vi "Main.vi"() -> ()   [LabVIEW 2023]
panel:
  in  "Marker_Size":string
  out "Color Box 5":u32(colorbox)
  out "Color Box 4":u32(colorbox)
  out "Color Box 3":u32(colorbox)
  out "Color Box 2":u32(colorbox)
  out "Color Box":u32(colorbox)
  out "error out":errorcluster
  out "Corner color":u32(colorbox)
  out "Colors traces":string
  out "standard output":string
  out "CLUT":u32[](array[numeric])
  in  "Path":path
  in  "style of points":string
  out "PnG picture":picture
  out "Pixmap vraie couleurs":u32[](array[numeric])
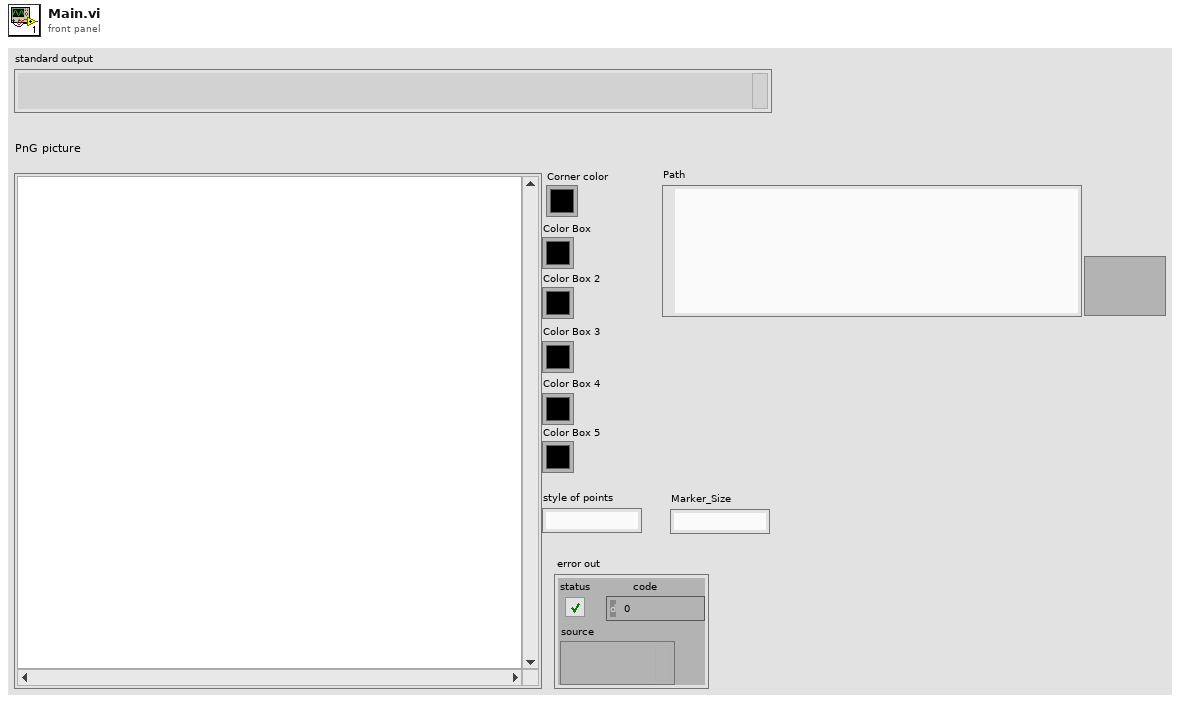
[diagram p1: front panel]
types:
  T1 = cluster{"[0]":u32, "[1]":u32, "[2]":u32, "[3]":u32, "[4]":u32, "[5]":u32, "[6]":u32, "[7]":u32, "[8]":u32}
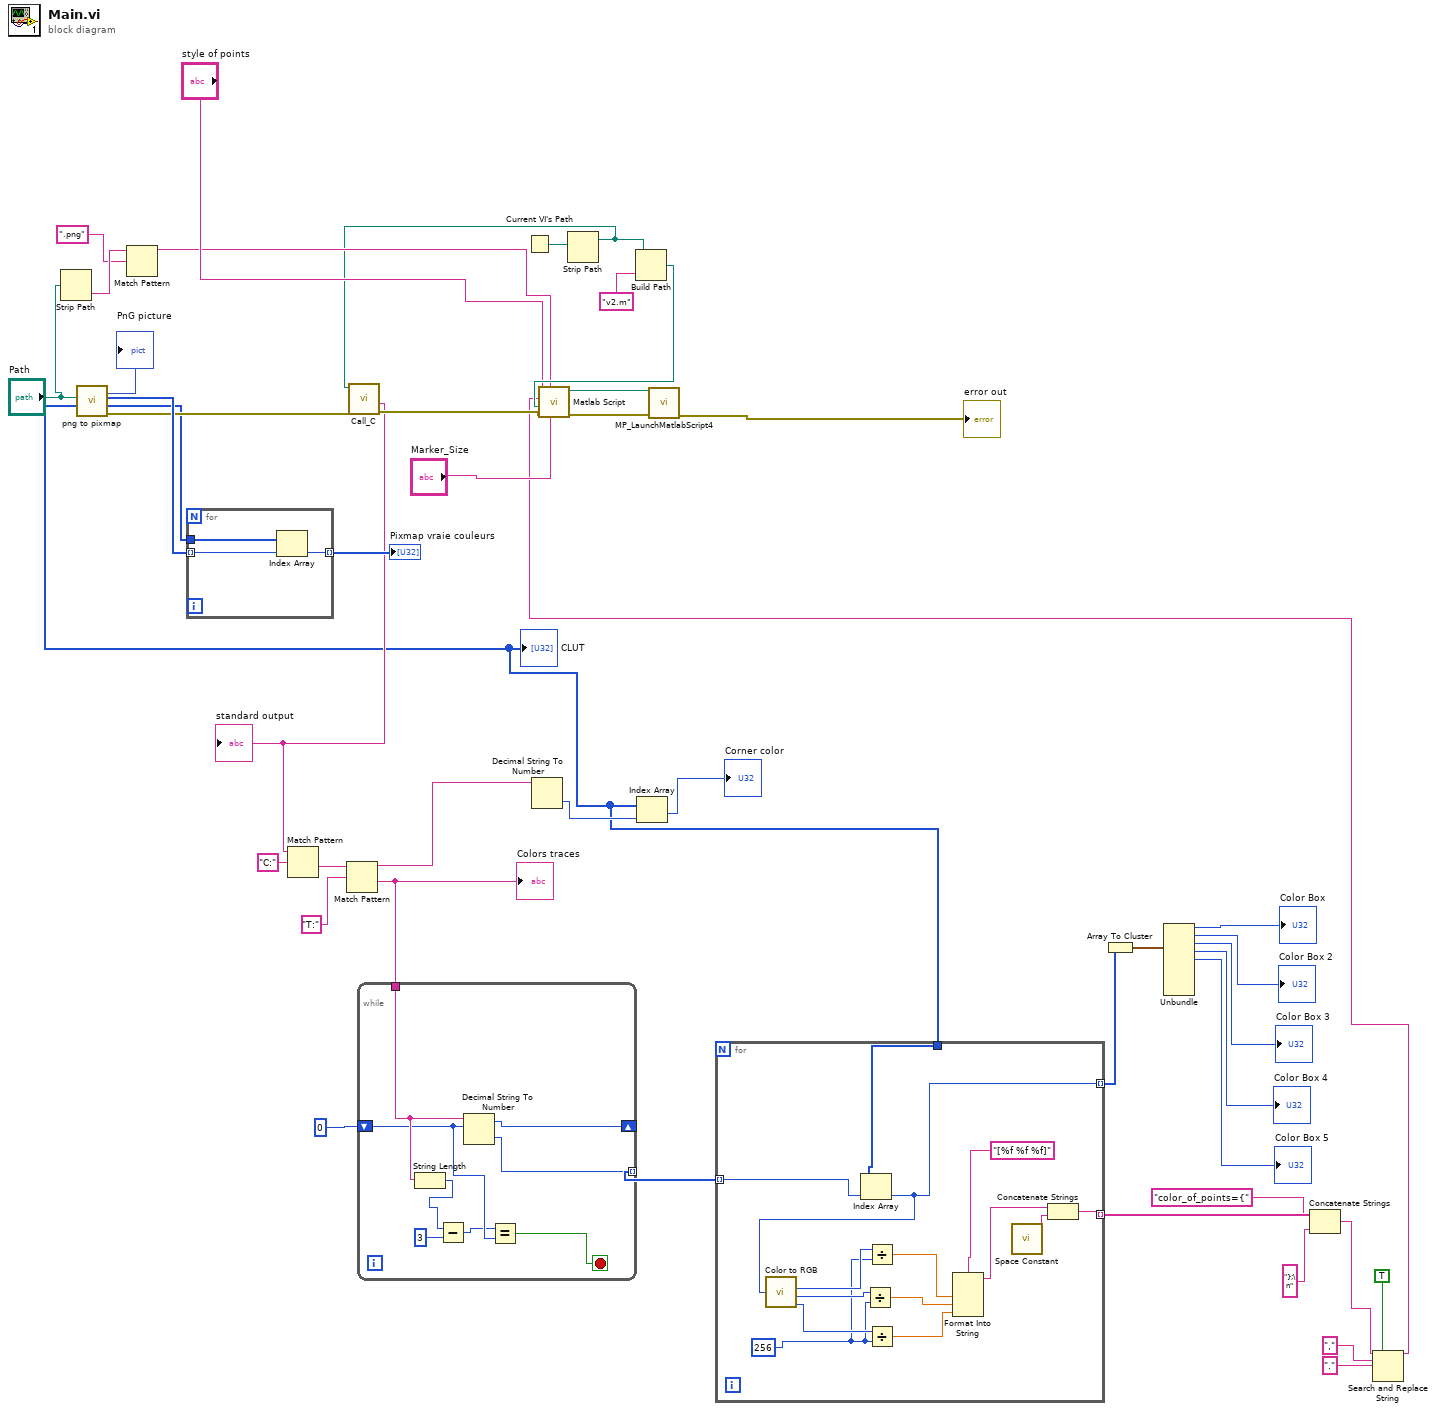
[diagram p0: block diagram]
diagram:
  n1 = Strip Path(path="Path") -> (name=w31:string)  [unwired: 1 out]
  n2 = call "png to pixmap.vi"("Path"="Path") -> ("error out"=w43:errorcluster, "Colors"=w20:u32[], "image"=w44:u8[], "PnG picture"=→"PnG picture":picture)  [unwired: 6 in, 1 out]
  "CLUT" <- w20
  n3 = Match Pattern(string=w31, regular expression=".png") -> (before substring=w29:string)  [unwired: 1 in, 3 out]
  n4 = for {
    tunnel: w44 -> [w46] mode=indexing
    tunnel: [w45] -> w34 mode=indexing
    tunnel: w20 -> [w47]
    n5 = Index Array(array=w47, index=w46) -> (element=w45:u32)
  }
  "Pixmap vraie couleurs" <- w34
  n6 = Current VI's Path() -> (path=w38:path)
  n7 = Strip Path(path=w38) -> (stripped path=w28:path)  [unwired: 1 out]
  n8 = call "Call_C.vi"("error in (no error)"=w43, "working directory"=w28) -> ("error out 2"=w42:errorcluster, "standard output"=w27:string)  [unwired: 7 in, 1 out]
  "standard output" <- w27
  n9 = Match Pattern(string=w27, regular expression="C:") -> (after substring=w25:string)  [unwired: 1 in, 3 out]
  n10 = Match Pattern(string=w25, regular expression="T:") -> (before substring=w23:string, after substring=w15:string)  [unwired: 1 in, 2 out]
  "Colors traces" <- w15
  n11 = while {
    shift-right: [w55] -> _
    shift-left: 0 -> [w51]
    tunnel: w15 -> [w53]
    tunnel: [w54] -> w14 mode=indexing
    stop <- w52 stop-if-true
    n12 = String Length(string=w53) -> (length=w50:i32)
    n13 = Subtract(x=w50, y=3) -> (x-y=w48:i32)
    n14 = Decimal String To Number(string=w53, offset=w51) -> (offset past number=w55:i32, number=w54:i32)  [unwired: 1 in]
    n15 = Equal?(x=w48, y=w51) -> (x = y?=w52:bool)
  }
  n16 = Decimal String To Number(string=w23) -> (number=w22:i32)  [unwired: 2 in, 1 out]
  n17 = Build Path(base path=w28, name or relative path="v2.m") -> (appended path=w36:path)
  n18 = Index Array(array=w20, index=w22) -> (element=→"Corner color":u32)
  n19 = for {
    tunnel: w20 -> [w69]
    tunnel: [w68] -> w19 mode=indexing
    tunnel: w14 -> [w67] mode=indexing
    tunnel: [w58] -> w13 mode=indexing
    w57 = 256
    n20 = Index Array(array=w69, index=w67) -> (element=w58:u32)
    n21 = call <vilib>:"Color to RGB.vi"("Color"=w58) -> ("R"=w60:u8, "G"=w61:u8, "B"=w62:u8)  [unwired: 1 out]
    n22 = Divide(x=w61, y=w57) -> (x/y=w64:dbl)
    n23 = Divide(x=w60, y=w57) -> (x/y=w63:dbl)
    n24 = Divide(x=w62, y=w57) -> (x/y=w65:dbl)
    n25 = Format Into String(format string="[%f %f %f]", w63, w64, w65) -> (resulting string=w59:string)  [unwired: 2 in, 1 out]
    n26 = call <vilib>:"Space Constant.vi"() -> ("String"=w66:string)
    n27 = Concatenate Strings(w59, w66) -> (w68:string)
  }
  n28 = Array To Cluster(array=w13) -> (cluster=w12:T1)
  n29 = Unbundle(w12) -> ("[0]"=→"Color Box":u32, "[1]"=→"Color Box 2":u32, "[2]"=→"Color Box 3":u32, "[3]"=→"Color Box 4":u32, "[4]"=→"Color Box 5":u32)  [unwired: 4 out]
  n30 = Concatenate Strings("color_of_points={" ("string"), w19, "};\n" ("string")) -> (w2:string)
  n31 = Search and Replace String(replace all?=TRUE ("replace all? (F)"), input string=w2, search string=",", replace string="." ("replace string (\"\")")) -> (result string=w1:string)  [unwired: 4 in, 3 out]
  n32 = call "Matlab Script.vi"("Marker_Size"="Marker_Size", "nom source"=w29, "error in"=w42, "path to matlab"=w36, "Color of points"=w1, "style of points"="style of points") -> ("error out"=w41:errorcluster, "path"=w40:path)  [unwired: 4 in]
  n33 = call "MP_LaunchMatlabScript4.vi"("error in (no error)"=w41, "matlab script path"=w40) -> ("error out"=→"error out":errorcluster)  [unwired: 4 in, 5 out]
